vi "MEASURE.vi"(7 "LabVIEW Web Service Request":refnum<class "Web Request.lvclass">, 10 "DURATION":u16, 11 "DEVICE_SN":string) -> ()   [LabVIEW 2015]
uses:
  <vilib>/wsapi/Web Request.lvclass
panel:
  # "Use the Web Service Request input terminal to call the VIs on the Web Services palette. Do not remove it from the connector pane unless you don't need access to the palette."
  # "Each additional control wired to the connector pane will be available as an input in the URL. To include an indicator in terminal-mode output (the default setting), it must also be wired to the connector pane."
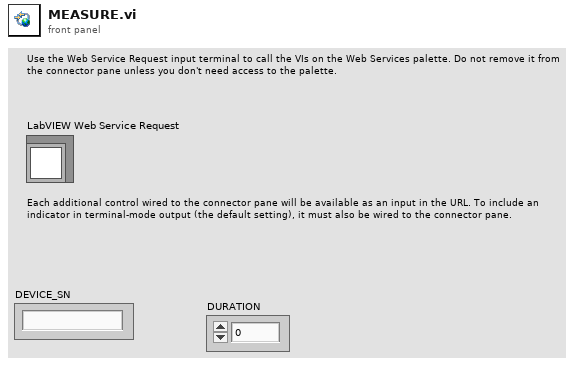
[diagram p1: front panel]
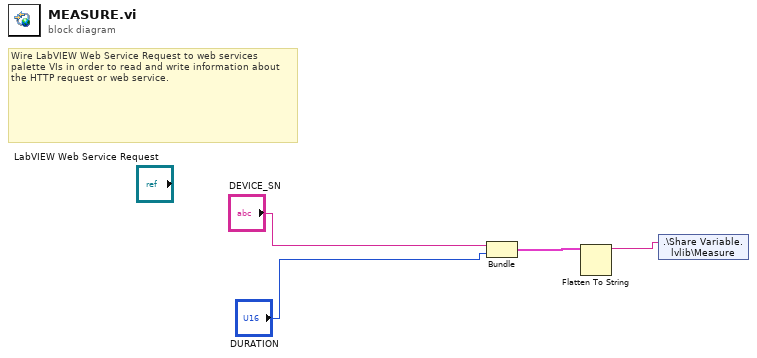
[diagram p0: block diagram]
diagram:
  # "Wire LabVIEW Web Service Request to web services palette VIs in order to read and write information about the HTTP request or web service."
  n1 = Bundle("DEVICE_SN"="DEVICE_SN", "DURATION"="DURATION") -> (w2:cluster{"DEVICE_SN":string, "DURATION":u16})  [unwired: 1 in]
  n2 = Flatten To String(anything=w2) -> (data string=w1:string)  [unwired: 3 in, 2 out]
  n3 = shared-variable ".\\Share Variable.lvlib\\Measure"(w1) -> ()  [unwired: 1 in, 1 out]
